vi "(Var) System.vi"() -> ()   [LabVIEW 2017]
panel:
  out "Exit":bool
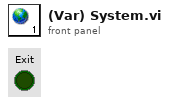
[diagram p1: front panel]
diagram:
